vi "Read.vi"(8 "error in (no error)":errorcluster, 9 "timeout ms (25000)":i32=2000, 11 "connection ID":refnum<k16>) -> (0 "error out":errorcluster, 2 "data out":string, 3 "connection ID":refnum<k16>, 4 "port":u16, 6 "address":u32)   [LabVIEW 2018, in "Simple UDP Message.lvlib"]
uses:
  Simple UDP Message.lvlib
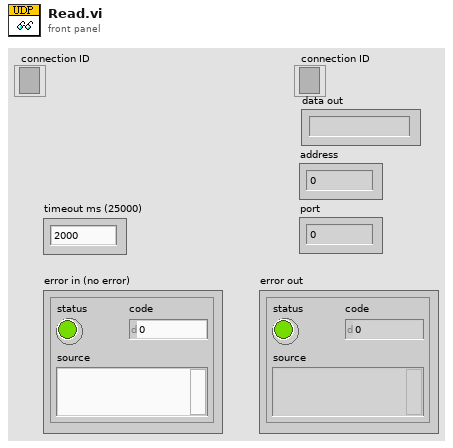
[diagram p1: front panel]
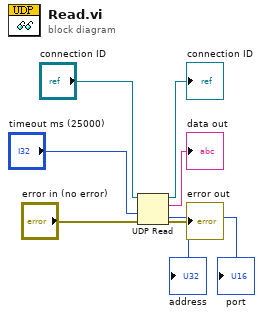
[diagram p0: block diagram]
diagram:
  n1 = UDP Read(connection ID="connection ID", timeout ms (25000)="timeout ms (25000)", 8:"error in (no error)") -> (data out=→"data out":string, error out=→"error out":errorcluster, 3:→"connection ID":refnum<k16>, 4:→"port":u16, 6:→"address":u32)  [unwired: 1 in]
